vi "Get-value-reference.vi"(8 "error in (no error)":errorcluster, 11 "Analysis params in":refnum<class "CV-Analysis.lvclass">) -> (0 "error out":errorcluster, 3 "Analysis params. ref.":refnum<data-value>)   [LabVIEW 2013, in "CameraVision.lvlib" / "CV-Analysis.lvclass"]
uses:
  CV-Analysis.lvclass
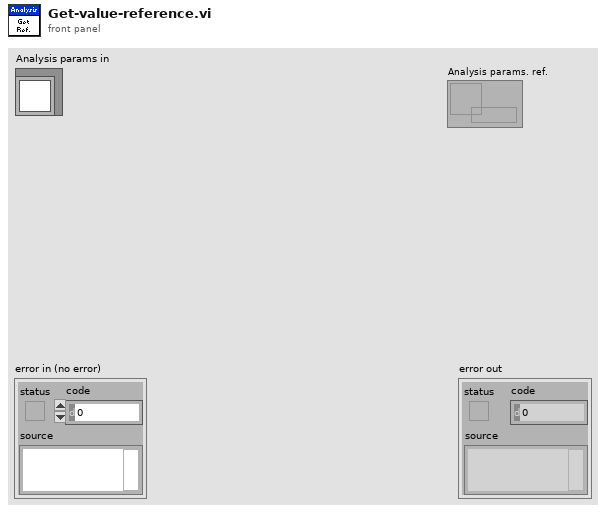
[diagram p1: front panel]
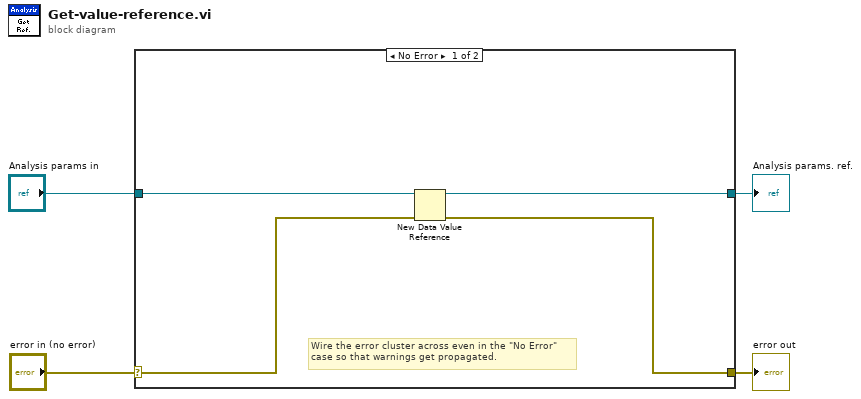
[diagram p0: block diagram]
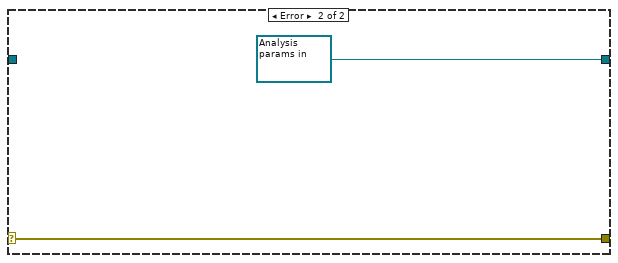
[diagram p2: hidden frame]
diagram:
  n1 = case shown="No Error" "error in (no error)" {
    selector: "error in (no error)" -> [w7 w10]
    tunnel: [w6 w10] -> w3
    tunnel: "Analysis params in" -> [w8 _]
    tunnel: [w5 refnum<data-value> refnum ("data value reference")] -> w1
    frame No Error {
      # "Wire the error cluster across even in the \"No Error\"\ncase so that warnings get propagated."
      n2 = New Data Value Reference(data value=w8, error in=w7) -> (data value reference=w5:refnum<data-value>, error out=w6:errorcluster)
    }
    frame Error {
    }
  }
  "error out" <- w3
  "Analysis params. ref." <- w1
